vi "SCMP - reverse array.vi"(11 "A in":u16[](array[numeric])) -> (3 "Array":u16[](array[numeric]))   [LabVIEW 2014]
panel:
  out "size / 2":i32
  out "size(s)":i32
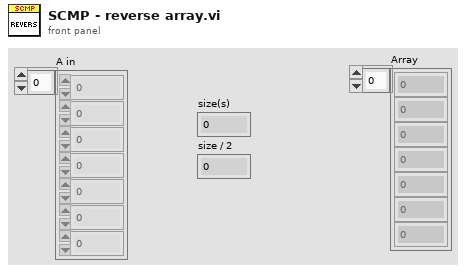
[diagram p1: front panel]
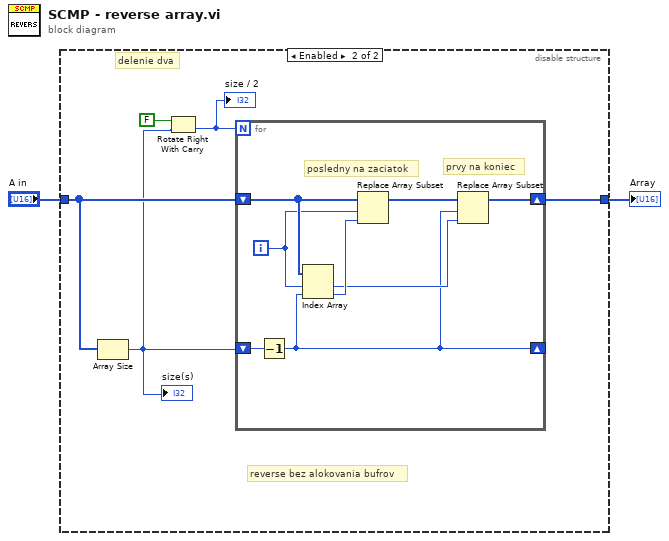
[diagram p0: block diagram]
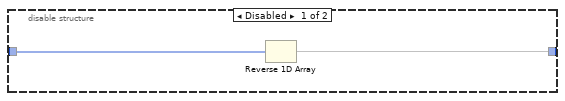
[diagram p2: hidden frame]
diagram:
  n1 = disable-structure shown="Enabled" {
    disable-tunnel: [w4 w8] -> w2
    disable-tunnel: "A in" -> [w3 w9]
    frame Disabled {
      n2 = Reverse 1D Array(array=w3) -> (reversed array=w4:u16[])
    }
    frame Enabled {
      # "reverse bez alokovania bufrov"
      # "delenie dva"
      n3 = Array Size(array=w9) -> (size(s)=w7:i32)
      "size(s)" <- w7
      n4 = Rotate Right With Carry(2:w7, 3:FALSE ("carry")) -> (0:w5:i32)  [unwired: 1 out]
      "size / 2" <- w5
      n5 = for {
        N: w5 -> [_]
        shift-right: [w13] -> w8
        shift-left: w9 -> [w17]
        shift-right: [w10] -> _
        shift-left: w7 -> [w11]
        i -> [w15]
        # "posledny na zaciatok"
        # "prvy na koniec"
        n6 = Decrement(x=w11) -> (x-1=w10:i32)
        n7 = Index Array(array=w17, index #1=w15, index #2=w10) -> (element #1=w12:u16, element #2=w16:u16)
        n8 = Replace Array Subset(array=w17, new element=w16, index=w15) -> (w14:u16[])
        n9 = Replace Array Subset(array=w14, new element=w12, index=w10) -> (w13:u16[])
      }
    }
  }
  "Array" <- w2
